vi "New.vi"(8 "error in (no error)":errorcluster, 11 "reference in":refnum<class "Bus Controller Suite.lvclass">) -> (0 "error out":errorcluster, 3 "reference out":refnum<class "Bus Controller Suite.lvclass">)   [LabVIEW 2016, in "Bus Controller Suite.lvclass"]
uses:
  Bus Controller Suite.lvclass
  D:/Programs/National Instruments/LabVIEW 2016/vi.lib/addons/_JKI Toolkits/VI Tester/TestSuite.llb/TestSuite.lvclass
  <vilib>/addons/_JKI Toolkits/VI Tester/TestCase.llb/TestCase.lvclass
  BC Async SubRoutines/BC Async SubRoutines.lvclass
  D:/SVN/Products/SLSC/Multichannel 1553 Module/Software/Source Code/Driver (Windows)/Unit Tests/1553 Test/1553 Test.lvclass
  BC Major Frame/BC Major Frame.lvclass
  BC Message/BC Message.lvclass
  BC Minor Frame/BC Minor Frame.lvclass
  BC Configuration/BC Configuration.lvclass
  1553 Test/1553 Test.lvclass
  D:/Programs/National Instruments/LabVIEW 2016/vi.lib/addons/_JKI Toolkits/VI Tester/TestCase.llb/TestCase.lvclass
  <vilib>/addons/_JKI Toolkits/VI Tester/TestSuite.llb/TestSuite.lvclass
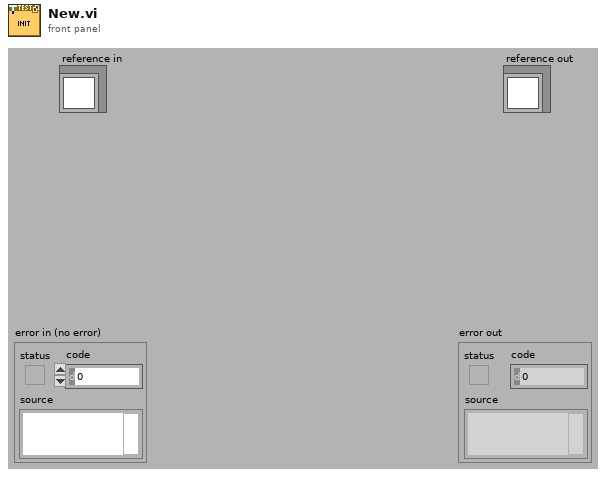
[diagram p1: front panel]
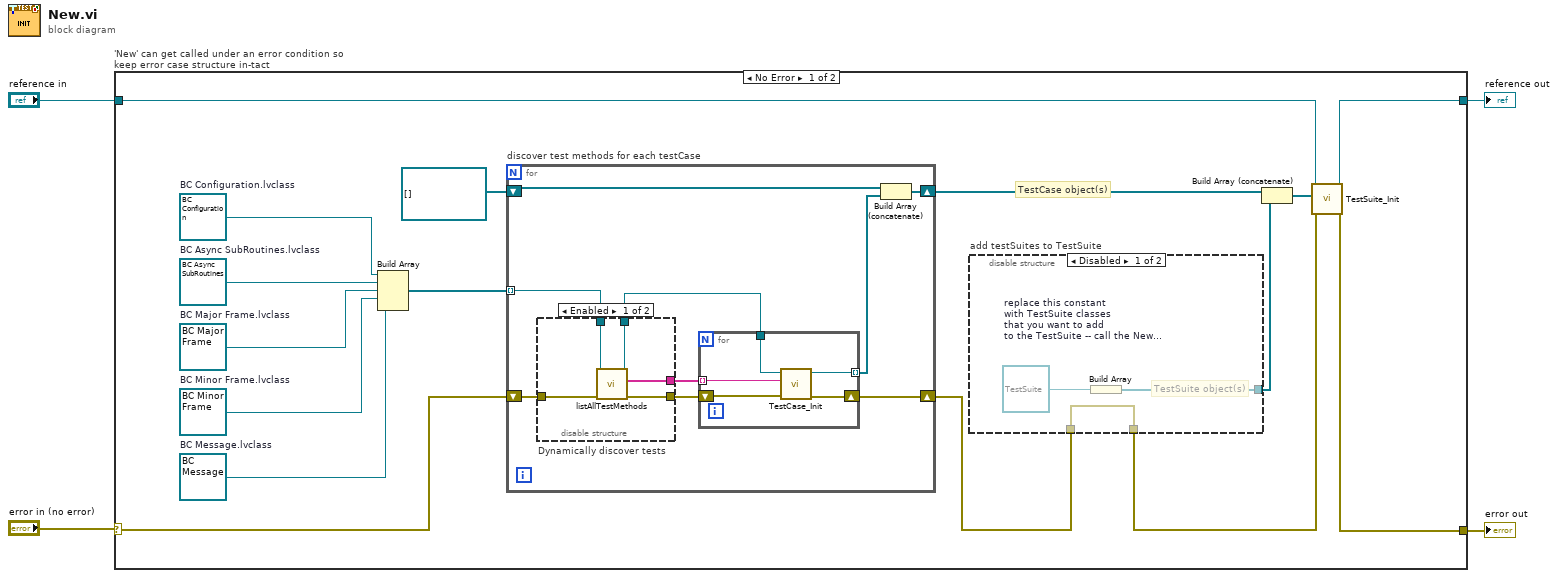
[diagram p0: block diagram]
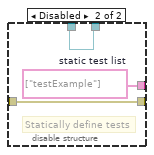
[diagram p2: hidden frame]
diagram:
  n1 = case "'New' can get called under an error condition so keep error case structure in-tact" shown="No Error" "error in (no error)" {
    selector: "error in (no error)" -> [w17 w47]
    tunnel: [w10 w48] -> w4
    tunnel: "reference in" -> [w18 w48]
    tunnel: [w20 w47] -> w1
    frame No Error {
      w5 = refnum<class "BC Configuration.lvclass"> refnum  # BC Configuration.lvclass
      w7 = refnum<class "BC Minor Frame.lvclass"> refnum  # BC Minor Frame.lvclass
      w6 = refnum<class "BC Message.lvclass"> refnum  # BC Message.lvclass
      w8 = refnum<class "BC Major Frame.lvclass"> refnum  # BC Major Frame.lvclass
      w9 = refnum<class "BC Async SubRoutines.lvclass"> refnum  # BC Async SubRoutines.lvclass
      # "TestCase object(s)"
      n2 = Build Array(w5, w9, w8, w7, w6) -> (w19:refnum<class "1553 Test.lvclass">[])
      n3 = for "discover test methods for each testCase" {
        shift-right: [w29] -> w12
        shift-left: w17 -> [w25]
        tunnel: w19 -> [w22] mode=indexing
        shift-right: [w26] -> w16
        shift-left: refnum<class "TestCase.lvclass">[] [] -> [w27]
        n4 = disable-structure "Dynamically discover tests" shown="Enabled" {
          disable-tunnel: w25 -> [w34 w35]
          disable-tunnel: [w33 w35] -> w24
          disable-tunnel: [w32 w36] -> w23
          disable-tunnel: w22 -> [w31 w37]
          disable-tunnel: [w30 w37] -> w21
          frame Enabled {
            n5 = call-dynamic "listAllTestMethods.vi"("error in (no error)"=w34, "TestCase in"=w31) -> ("error out"=w33:errorcluster, "test methods"=w32:string[], "TestCase out"=w30:refnum<class "1553 Test.lvclass">)  [unwired: 7 in]
          }
          frame Disabled {
            w36 = string[] ["testExample"]  # static test list
            # "Statically define tests"
          }
        }
        n6 = for {
          tunnel: w21 -> [w38]
          tunnel: w23 -> [w42] mode=indexing
          shift-right: [w40] -> w29
          shift-left: w24 -> [w41]
          tunnel: [w39] -> w28 mode=indexing
          n7 = call <vilib>:"TestCase_Init.vi"("error in (no error)"=w41, "methodName (\"runTest\")"=w42, "TestCase in"=w38) -> ("error out"=w40:errorcluster, "TestCase out"=w39:refnum<class "1553 Test.lvclass">)  [unwired: 7 in]
        }
        n8 = Build Array (concatenate)(w27, w28) -> (w26:refnum<class "TestCase.lvclass">[])
      }
      n9 = disable-structure "add testSuites to TestSuite" shown="Disabled" {
        disable-tunnel: [w43 _] -> w14
        disable-tunnel: [w45 w46] -> w13
        disable-tunnel: w12 -> [w45 w46]
        frame Disabled {
          w44 = refnum<class "TestSuite.lvclass"> refnum  # replace this constant with TestSuite classes that you want to add to the TestSuite -- call the New method for each TestSuite prior to adding it to this TestSuite
          # "TestSuite object(s)"
          n10 = Build Array(w44) -> (w43:refnum<class "TestSuite.lvclass">[])
        }
        frame Enabled {
          # "by default, no TestSuites are defined\nas members of a TestSuite"
        }
      }
      n11 = Build Array (concatenate)(w16, w14) -> (w15:refnum<class>[])
      n12 = call <vilib>:"TestSuite_Init.vi"("error in (no error)"=w13, "tests (none)"=w15, "TestSuite in"=w18) -> ("error out"=w20:errorcluster, "TestSuite out"=w10:refnum<class "Bus Controller Suite.lvclass">)  [unwired: 7 in]
    }
    frame Error {
    }
  }
  "reference out" <- w4
  "error out" <- w1
